vi "TH_MakeLoadFilenames.vi"(7 "Input Dates":T1) -> (3 "Filenames":string[](array[string]))   [LabVIEW 2014]
panel:
  out "Size":dbl
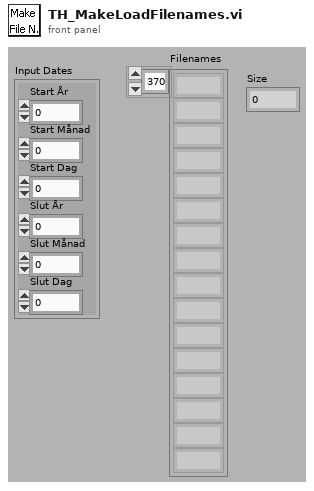
[diagram p1: front panel]
types:
  T1 = cluster{"Start År":u16, "Start Månad":u16, "Start Dag":u16, "Slut År":u16, "Slut Månad":u16, "Slut Dag":u16}
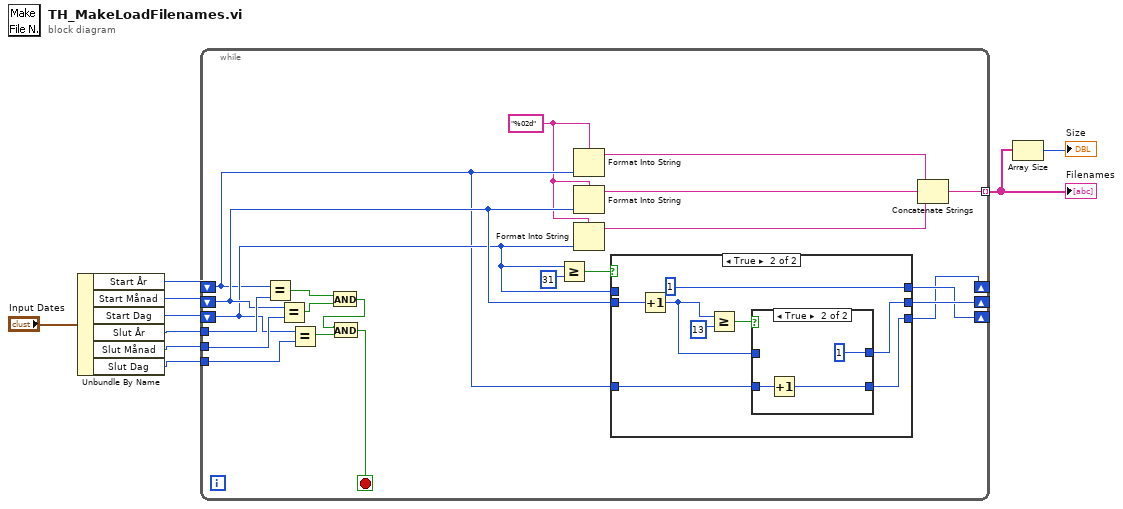
[diagram p0: block diagram]
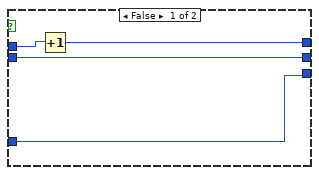
[diagram p2: hidden frame]
diagram:
  n1 = Unbundle By Name("Input Dates") -> ("Start År"=w5:u16, "Start Månad"=w4:u16, "Start Dag"=w3:u16, "Slut År"=w8:u16, "Slut Månad"=w7:u16, "Slut Dag"=w6:u16)
  n2 = while {
    tunnel: [w19] -> w1 mode=indexing
    shift-left: w3 -> [w14]
    shift-right: [w11] -> _
    shift-left: w4 -> [w16]
    shift-right: [w15] -> _
    shift-left: w5 -> [w13]
    shift-right: [w10] -> _
    tunnel: w6 -> [w28]
    tunnel: w7 -> [w29]
    tunnel: w8 -> [w30]
    stop <- w23 stop-if-true
    w12 = "%02d" ("Format String")
    n3 = Equal?(x=w13, y=w30) -> (x = y?=w27:bool)
    n4 = Equal?(x=w16, y=w29) -> (x = y?=w26:bool)
    n5 = Equal?(x=w14, y=w28) -> (x = y?=w25:bool)
    n6 = And(x=w27, y=w26) -> (x .and. y?=w24:bool)
    n7 = And(x=w24, y=w25) -> (x .and. y?=w23:bool)
    n8 = Greater Or Equal?(x=w14, y=u16 31) -> (x >= y?=w17:bool)
    n9 = Format Into String(format string=w12, w13) -> (resulting string=w22:string)  [unwired: 2 in, 1 out]
    n10 = Format Into String(format string=w12, w16) -> (resulting string=w20:string)  [unwired: 2 in, 1 out]
    n11 = Format Into String(format string=w12, w14) -> (resulting string=w21:string)  [unwired: 2 in, 1 out]
    n12 = case shown="True" w17 {
      tunnel: w16 -> [w34 w42]
      tunnel: [w34 w36] -> w15
      tunnel: [w33 1] -> w11
      tunnel: w14 -> [w32 _]
      tunnel: w13 -> [w31 w38]
      tunnel: [w31 w35] -> w10
      frame False {
        n13 = Increment(x=w32) -> (x+1=w33:i32)
      }
      frame True {
        n14 = Increment(x=w42) -> (x+1=w37:i32)
        n15 = Greater Or Equal?(x=w37, y=u16 13) -> (x >= y?=w39:bool)
        n16 = case shown="True" w39 {
          tunnel: w38 -> [w43 w47]
          tunnel: w37 -> [w44 _]
          tunnel: [w44 1] -> w36
          tunnel: [w43 w45] -> w35
          frame False {
          }
          frame True {
            n17 = Increment(x=w47) -> (x+1=w45:u16)
          }
        }
      }
    }
    n18 = Concatenate Strings(w22, w20, w21) -> (w19:string)
  }
  "Filenames" <- w1
  n19 = Array Size(array=w1) -> (size(s)=→"Size":i32)
